vi "LV to ITX 2.2 ITX2.vi"(0 "Commands":string, 5 "filename":path, 7 "Notes":string, 8 "wavenames":string[](array[string]), 9 "array of clusters":cluster{"Y  Array":dbl[]}[](array[cluster])) -> (3 "file":path)   [LabVIEW 2013]
panel:
  out "String":string
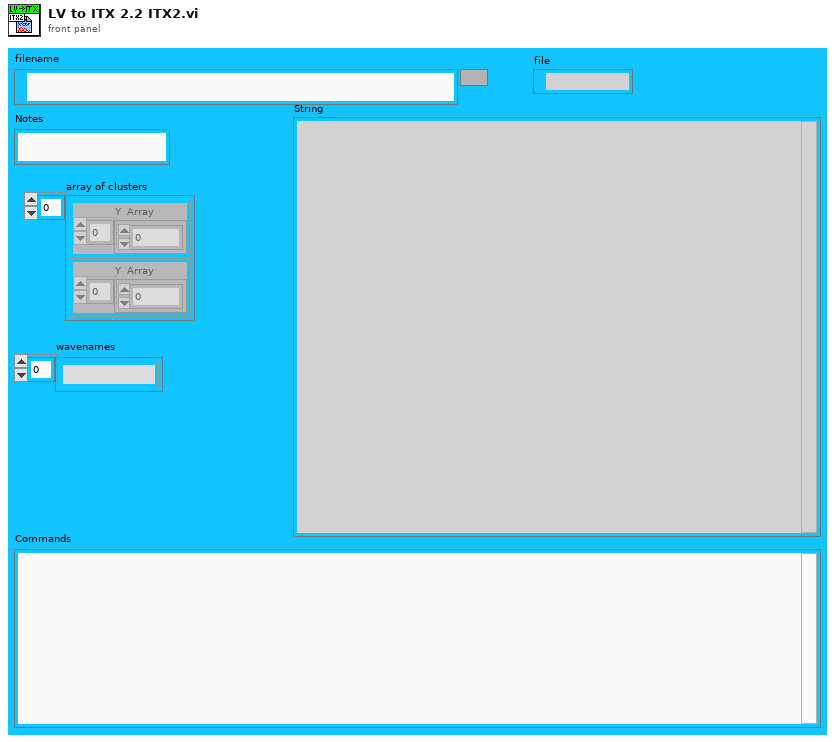
[diagram p1: front panel]
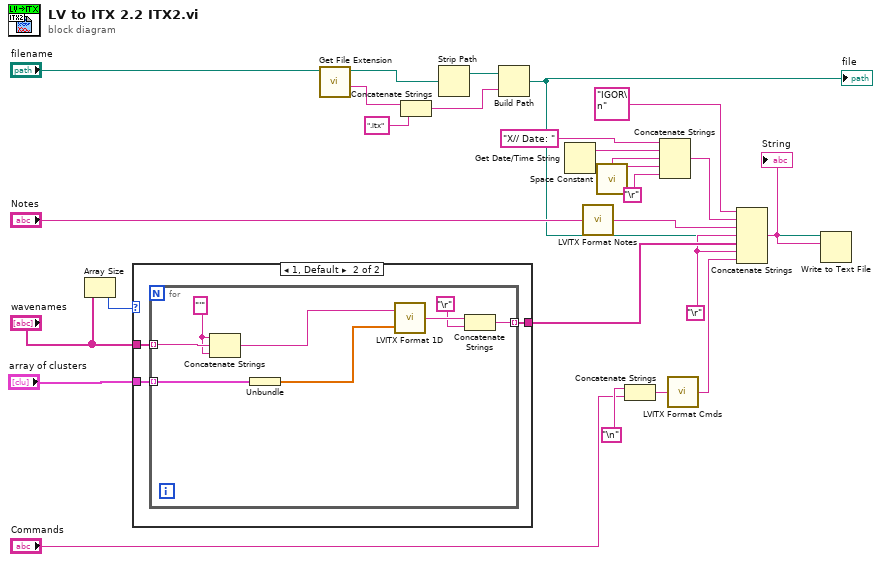
[diagram p0: block diagram]
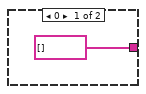
[diagram p2: hidden frame]
diagram:
  w7 = "\r"
  n1 = Array Size(array="wavenames") -> (size(s)=w11:i32)
  n2 = case shown="1, Default" w11 {
    tunnel: "wavenames" -> [_ w30]
    tunnel: "array of clusters" -> [_ w29]
    tunnel: [string[] [] w28] -> w14
    frame 0 {
    }
    frame 1, Default {
      n3 = for {
        tunnel: [w38] -> w28 mode=indexing
        tunnel: w30 -> [w34] mode=indexing
        tunnel: w29 -> [w35] mode=indexing
        w32 = "'"
        n4 = Concatenate Strings(w32, w34, w32) -> (w31:string)
        n5 = Unbundle(w35) -> ("Y  Array"=w33:dbl[])
        n6 = call "LVITX Format 1D.vi"("X 1D Array"=w33, "X  Array name"=w31) -> ("String"=w37:string)
        n7 = Concatenate Strings(w37, "\r") -> (w38:string)
      }
    }
  }
  n8 = call <vilib>:"Get File Extension.vi"("file"="filename") -> ("filename without extension"=w21:string, "dup file"=w18:path)  [unwired: 1 in, 8 out]
  n9 = Concatenate Strings(w21, ".itx") -> (w16:string)
  n10 = Strip Path(path=w18) -> (stripped path=w17:path)  [unwired: 1 out]
  n11 = Build Path(base path=w17, name or relative path=w16) -> (appended path=w3:path)
  "file" <- w3
  n12 = Get Date/Time String() -> (date string=w25:string, time string=w26:string)  [unwired: 3 out]
  n13 = call "LVITX Format Notes.vi"("Notes"="Notes") -> ("String"=w4:string)
  n14 = call <vilib>:"Space Constant.vi"() -> ("String"=w23:string)
  n15 = Concatenate Strings("\n", "Commands") -> (w19:string)
  n16 = Concatenate Strings("X// Date: " ("format string"), w25, w23, w26, "\r") -> (w6:string)
  n17 = call "LVITX Format Cmds.vi"("Commands"=w19) -> ("String"=w1:string)
  n18 = Concatenate Strings("IGOR\n", w6, w4, w7, w14, w7, w1) -> (w13:string)
  "String" <- w13
  n19 = Write to Text File(file (use dialog)=w3, text=w13) -> ()  [unwired: 1 in, 4 out]
